vi "Filter or Update Disabled Forecasts by ID.vi"(8 "error in":errorcluster, 11 "Generic Optimization in":refnum<class "Generic Optimization.lvclass">) -> (0 "dup error out":errorcluster, 3 "Generic Optimization out":refnum<class "Generic Optimization.lvclass">)   [LabVIEW 2018, in "Generic Optimization Actor.lvlib" / "Generic Optimization.lvclass"]
uses:
  Generic Optimization.lvclass
  C:/Users/Administrator/Desktop/2018LabVIEW EMS/EMS Generic Actor/EMS Generic/EMS Generic.lvclass
  EMS Generic Actor/EMS Generic/EMS Generic.lvclass/EMS Generic.ctl
  <vilib>/ORNL/CSEISMIC DDS/CSEISMIC DDS Base/Data Types/IED_Status.ctl
  <vilib>/ORNL/CSEISMIC DDS/CSEISMIC DDS Base/Data Types/Controls/DeviceID.ctl
  <vilib>/ORNL/CSEISMIC DDS/CSEISMIC DDS Base/Data Types/Controls/Timestamp.ctl
  <vilib>/ORNL/CSEISMIC DDS/CSEISMIC DDS Base/Data Types/Controls/DeviceClass Selector.ctl
  <vilib>/ORNL/CSEISMIC DDS/CSEISMIC DDS Base/Data Types/PriceData_RealTime.ctl
  <vilib>/ORNL/CSEISMIC DDS/CSEISMIC DDS Base/Data Types/ForecastData_Data.ctl
  EMS Generic Actor/EMS Generic/EMS Generic.lvclass
  <vilib>/ORNL/CSEISMIC DDS/CSEISMIC DDS Base/CSEISMIC DDS.lvclass
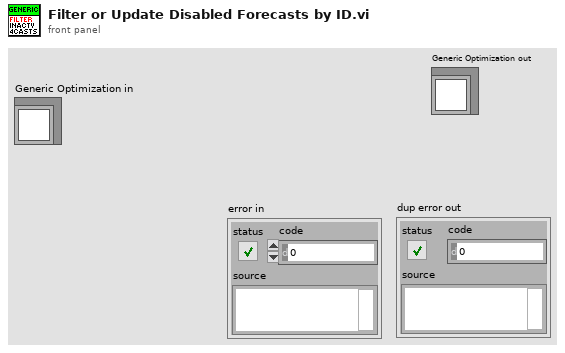
[diagram p1: front panel]
types:
  T1 = typedef "EMS Generic Actor.lvlib/EMS Generic.lvclass/Data Type DVRs.ctl" = cluster{"IED_Status":refnum<data-value>, "IED_Status_0":refnum<data-value>, "DER_Measurement":refnum<data-value>, "DER_Info":refnum<data-value>, "DER_Status":refnum<data-value>, "ES_Measurement":refnum<data-value>, "ES_Info":refnum<data-value>, "PV_Info":refnum<data-value>, "SmartRelay_Info":refnum<data-value>, "SmartRelay_Measurement":refnum<data-value>, "Meter_Info":refnum<data-value>, "Meter_Measurement":refnum<data-value>, "HVAC_Status":refnum<data-value>, "HVAC_Measurement":refnum<data-value>, "PriceData_RealTime":refnum<data-value>, "PriceData_Demand":refnum<data-value>, "PriceData_Energy":refnum<data-value>, "ForecastData_Long":refnum<data-value>, "ForecastData_Short":refnum<data-value>, "DER_Control":refnum<data-value>, "DER_SetPointF":refnum<data-value>, "DER_SetPointP":refnum<data-value>, "DER_SetPointQ":refnum<data-value>, "DER_SetPointPF":refnum<data-value>, "DER_SetPointV":refnum<data-value>, "PV_setCurtailment":refnum<data-value>, "PV_setRampRate":refnum<data-value>, "Relay_Control":refnum<data-value>, "Load_Control":refnum<data-value>, "HVAC_Control":refnum<data-value>, "Generator_Info":refnum<data-value>, "ForecastData_Long_Backup":refnum<data-value>, "PriceData_RealTime_Backup":refnum<data-value>}
  T2 = typedef "CSEISMIC DDS.lvlib/CSEISMIC DDS.lvclass/IED_Status.ctl" = cluster{"DeviceID":T3, "Timestamp":T4, "MicrogridID":u8, "Active":bool, "Inactive":bool, "Error":i32, "Fault":bool, "ErrorString":string}
  T3 = typedef "CSEISMIC DDS.lvlib/CSEISMIC DDS.lvclass/DeviceID.ctl" = string
  T4 = typedef "CSEISMIC DDS.lvlib/CSEISMIC DDS.lvclass/Timestamp.ctl" = cluster{"Seconds":u64, "Remainder":u64}
  T5 = typedef "CSEISMIC DDS.lvlib/CSEISMIC DDS.lvclass/PriceData_RealTime.ctl" = cluster{"DeviceID":T3, "t0":dbl, "dt":dbl, "Price":dbl[]}
  T6 = typedef "CSEISMIC DDS.lvlib/CSEISMIC DDS.lvclass/ForecastData_Data.ctl" = cluster{"DeviceID":T3, "TargetID":T3, "t0":dbl, "dt":dbl, "Magnitude":dbl[]}
  T7 = typedef "CSEISMIC DDS.lvlib/CSEISMIC DDS.lvclass/DeviceClass Selector.ctl" = u16
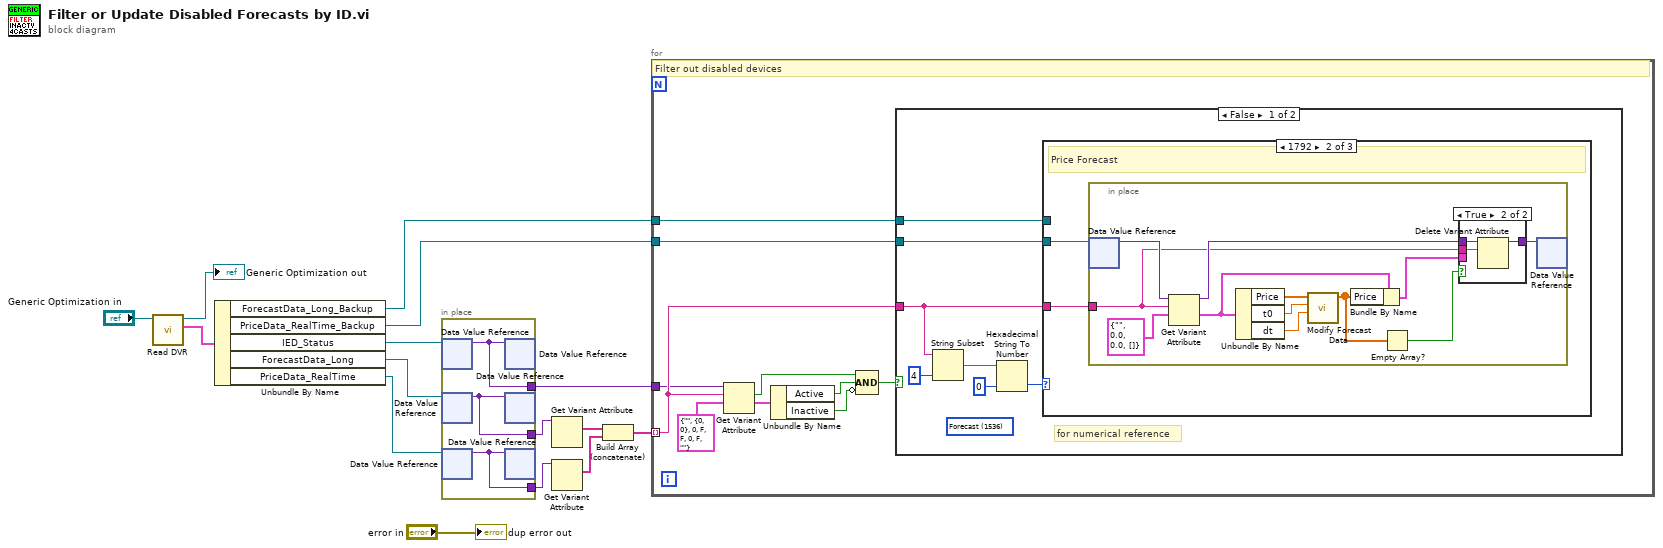
[diagram p0: block diagram]
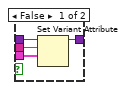
[diagram p3: hidden frame]
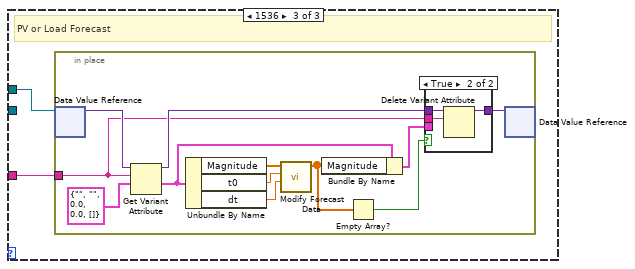
[diagram p4: hidden frame]
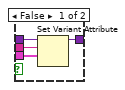
[diagram p5: hidden frame]
diagram:
  n1 = call "Read DVR.vi"("EMS Generic in"="Generic Optimization in") -> ("DVR"=w13:T1, "EMS Generic out"=→"Generic Optimization out":refnum<class "Generic Optimization.lvclass">)  [unwired: 9 in]
  n2 = Unbundle By Name(w13) -> ("ForecastData_Long_Backup"=w8:refnum<data-value>, "PriceData_RealTime_Backup"=w9:refnum<data-value>, "IED_Status"=w14:refnum<data-value>, "ForecastData_Long"=w7:refnum<data-value>, "PriceData_RealTime"=w6:refnum<data-value>)
  n3 = in-place {
    in-place-border: [w18] -> w15
    in-place-border: [w17] -> w5
    in-place-border: [w16] -> w4
    n4 = in-place-dvr #1(w14) -> (w18:variant)  [unwired: 1 out]
    n5 = in-place-dvr #2(w7) -> (w17:variant)  [unwired: 1 out]
    n6 = in-place-dvr #3(w6) -> (w16:variant)  [unwired: 1 out]
    n7 = in-place-dvr #1(w18) -> ()  [unwired: 2 out]
    n8 = in-place-dvr #2(w17) -> ()  [unwired: 2 out]
    n9 = in-place-dvr #3(w16) -> ()  [unwired: 2 out]
  }
  n10 = Get Variant Attribute(Variant=w5) -> (names=w3:string[])  [unwired: 3 in, 3 out]
  n11 = Get Variant Attribute(Variant=w4) -> (names=w2:string[])  [unwired: 3 in, 3 out]
  n12 = Build Array (concatenate)(w3, w2) -> (w1:string[])
  n13 = for {
    tunnel: w1 -> [w28] mode=indexing
    tunnel: w15 -> [w22]
    tunnel: w9 -> [w24]
    tunnel: w8 -> [w23]
    # "Filter out disabled devices"
    n14 = Get Variant Attribute(Variant=w22, name=w28, default value (empty Variant)=T2 {"DeviceID"="", "Timestamp"={"Seconds"=0, "Remainder"=0}, "MicrogridID"=0, "Active"=FALSE, "Inactive"=FALSE, "Error"=0, "Fault"=FALSE, "ErrorString"=""} ("IED_Status")) -> (found=w19:bool, value=w20:T2)  [unwired: 1 in, 2 out]
    n15 = Unbundle By Name(w20) -> ("Active"=w27:bool, "Inactive"=w26:bool)
    n16 = Compound Arithmetic op=AND(w19, w27, invert w26) -> (w25:bool)
    n17 = case shown="False" w25 {
      tunnel: w28 -> [w29 _]
      tunnel: w24 -> [w31 _]
      tunnel: w23 -> [w30 _]
      frame False {
        (unwired) T7 1536 items=["Invalid"=0, "IED"=256, "DER"=512, "Relay"=768, "Meter"=1024, "Load"=1280, "Forecast"=1536, "Price"=1792, "Energy Storage"=513, "PV"=514, "Generator"=515, "Smart Relay"=769, "PCC"=770, "Smart Meter"=1025, "PMU"=1026, "HVAC"=1281] ("DeviceClass")
        # "for numerical reference"
        n18 = String Subset(string=w29, length (rest)=4 ("length (rest)")) -> (substring=w34:string)  [unwired: 1 in]
        n19 = Hexadecimal String To Number(string=w34, default (0uL)=u16 0 ("default (0 U32)")) -> (number=w32:u16)  [unwired: 1 in, 1 out]
        n20 = case shown="1792" w32 {
          tunnel: w31 -> [_ w37 _]
          tunnel: w30 -> [_ _ w57]
          tunnel: w29 -> [_ w36 w58]
          frame 0, Default {
            # "Not a forecast"
          }
          frame 1792 {
            # "Price Forecast"
            n21 = in-place {
              in-place-border: w36 -> [w39]
              n22 = in-place-dvr #4(w37) -> (w46:variant)  [unwired: 1 out]
              n23 = Get Variant Attribute(Variant=w46, name=w39, default value (empty Variant)=T5 {"DeviceID"="", "t0"=0.0, "dt"=0.0, "Price"=[]} ("PriceData_RealTime")) -> (duplicate Variant=w42:variant, value=w44:T5)  [unwired: 1 in, 2 out]
              n24 = Unbundle By Name(w44) -> ("Price"=w49:dbl[], "t0"=w48:dbl, "dt"=w47:dbl)
              n25 = call "Modify Forecast Data.vi"("dt (sec)"=w47, "t0 (sec)"=w48, "array"=w49) -> ("Data"=w43:dbl[])  [unwired: 7 in, 1 out]
              n26 = Bundle By Name(cluster=w44, "Price"=w43) -> (w40:T5)
              n27 = Empty Array?(array=w43) -> (empty?=w38:bool)
              n28 = case shown="True" w38 {
                tunnel: w42 -> [w53 w55]
                tunnel: [w52 w56] -> w41
                tunnel: w40 -> [w51 _]
                tunnel: w39 -> [w50 w54]
                frame False {
                  n29 = Set Variant Attribute(Variant=w53, name=w50, value=w51) -> (Variant out=w52:variant)  [unwired: 1 in, 2 out]
                }
                frame True {
                  n30 = Delete Variant Attribute(6:w54, 7:w55) -> (3:w56:variant)  [unwired: 1 in, 2 out]
                }
              }
              n31 = in-place-dvr #4(w41) -> ()  [unwired: 2 out]
            }
          }
          frame 1536 {
            # "PV or Load Forecast"
            n32 = in-place {
              in-place-border: w58 -> [w62]
              n33 = in-place-dvr #5(w57) -> (w67:variant)  [unwired: 1 out]
              n34 = Get Variant Attribute(Variant=w67, name=w62, default value (empty Variant)=T6 {"DeviceID"="", "TargetID"="", "t0"=0.0, "dt"=0.0, "Magnitude"=[]} ("ForecastData")) -> (duplicate Variant=w65:variant, value=w66:T6)  [unwired: 1 in, 2 out]
              n35 = Unbundle By Name(w66) -> ("Magnitude"=w70:dbl[], "t0"=w69:dbl, "dt"=w68:dbl)
              n36 = call "Modify Forecast Data.vi"("dt (sec)"=w68, "t0 (sec)"=w69, "array"=w70) -> ("Data"=w60:dbl[])  [unwired: 7 in, 1 out]
              n37 = Bundle By Name(cluster=w66, "Magnitude"=w60) -> (w63:T6)
              n38 = Empty Array?(array=w60) -> (empty?=w59:bool)
              n39 = case shown="True" w59 {
                tunnel: w65 -> [w74 w76]
                tunnel: [w73 w77] -> w64
                tunnel: w63 -> [w72 _]
                tunnel: w62 -> [w71 w75]
                frame False {
                  n40 = Set Variant Attribute(Variant=w74, name=w71, value=w72) -> (Variant out=w73:variant)  [unwired: 1 in, 2 out]
                }
                frame True {
                  n41 = Delete Variant Attribute(6:w75, 7:w76) -> (3:w77:variant)  [unwired: 1 in, 2 out]
                }
              }
              n42 = in-place-dvr #5(w64) -> ()  [unwired: 2 out]
            }
          }
        }
      }
      frame True {
      }
    }
  }
  "dup error out" <- "error in"
